vi "环境参数上传.vi"(11 "错误输入（无错误）":errorcluster) -> (15 "error out":errorcluster)   [LabVIEW 2016, in "数据传输系统-04.lvlib"]
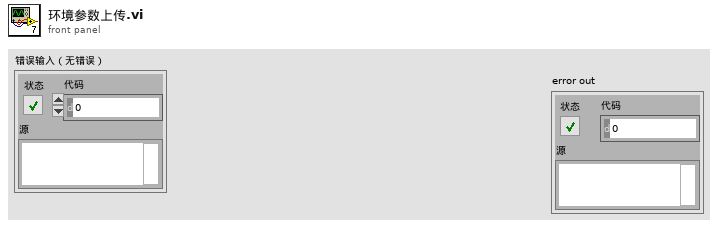
[diagram p1: front panel]
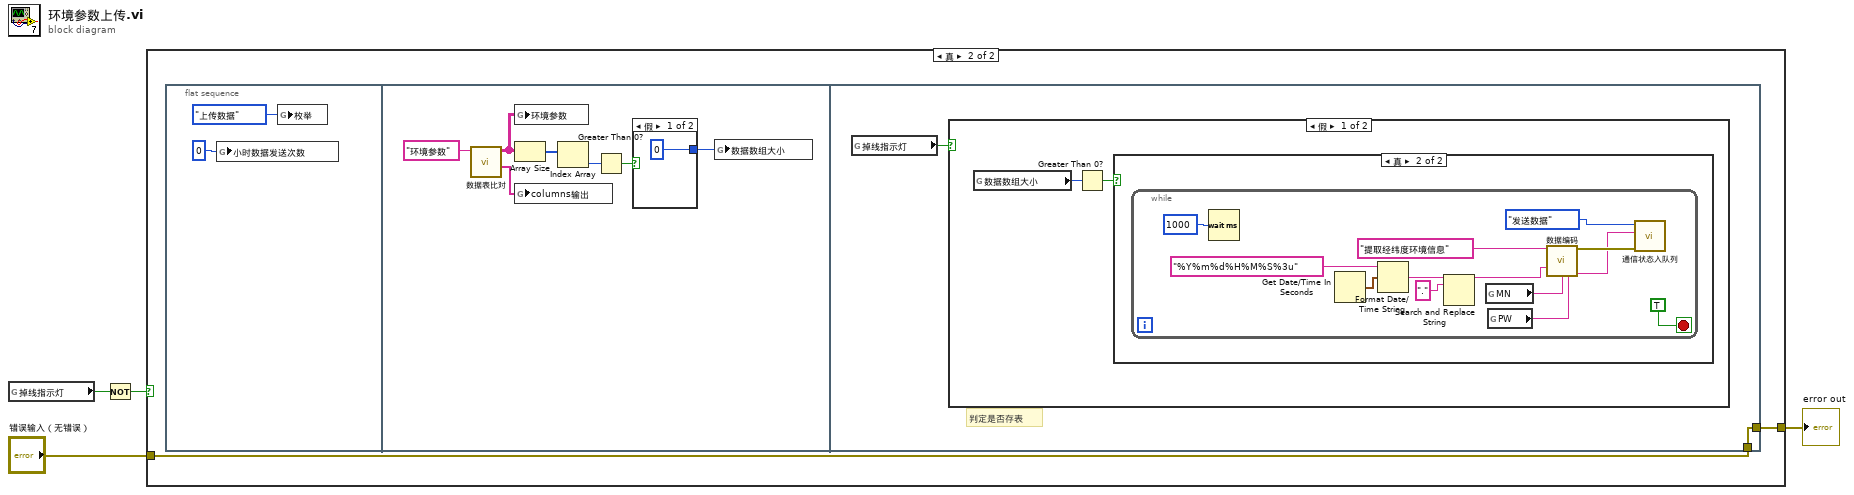
[diagram p0: block diagram]
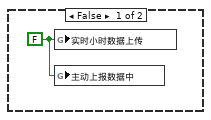
[diagram p2: hidden frame]
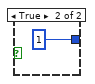
[diagram p3: hidden frame]
diagram:
  n1 = global read "全局 数据发送重叠.vi" "掉线指示灯"() -> (w4:bool)
  n2 = Not(x=w4) -> (.not. x?=w1:bool)
  n3 = case shown="真" w1 {
    tunnel: [_ w6] -> w3
    tunnel: "错误输入（无错误）" -> [_ w7]
    frame False {
      w5 = FALSE ("小时数据上传")
      n4 = global write "全局1.vi" "实时小时数据上传"(w5) -> ()
      n5 = global write "全局 数据发送重叠.vi" "主动上报数据中"(w5) -> ()
    }
    frame True {
      n6 = flat-sequence {
        tunnel: [w19] -> w6
        tunnel: w7 -> [w19]
        frame #0 {
          n7 = global write "全局 小时数据发送次数.vi" "小时数据发送次数"(0 ("小时数据发送次数")) -> ()
          n8 = global write "全局1.vi" "枚举"(enum16{"返回请求应答", "上传数据", "返回执行结果"}."上传数据" ("枚举")) -> ()
        }
        frame #1 {
          n9 = call "数据表比对.vi"("table输入"="环境参数" ("新元素/子数组")) -> ("columns输出"=w16:string[], "待发送数据"=w14:string[][])  [unwired: 7 in, 2 out]
          n10 = global write "全局 环境参数.vi" "环境参数"(w14) -> ()
          n11 = Array Size(array=w14) -> (size(s)=w13:i32[])
          n12 = global write "全局 环境参数.vi" "columns输出"(w16) -> ()
          n13 = Index Array(array=w13) -> (element=w12:i32)  [unwired: 1 in]
          n14 = Greater Than 0?(x=w12) -> (x > 0?=w11:bool)
          n15 = case shown="假" w11 {
            tunnel: [0 ("数据数组大小") 1 ("数据数组大小")] -> w10
            frame False {
            }
            frame True {
            }
          }
          n16 = global write "全局 数据数组大小.vi" "数据数组大小"(w10) -> ()
        }
        frame #2 {
          # "判定是否存表"
          n17 = global read "全局 数据发送重叠.vi" "掉线指示灯"() -> (w20:bool)
          n18 = case shown="假" w20 {
            frame False {
              n19 = global read "全局 数据数组大小.vi" "数据数组大小"() -> (w21:i32)
              n20 = Greater Than 0?(x=w21) -> (x > 0?=w22:bool)
              n21 = case shown="真" w22 {
                frame False {
                }
                frame True {
                  n22 = while {
                    stop <- TRUE stop-if-true
                    n23 = Wait (ms)(milliseconds to wait=u32 1000 ("等待时间（毫秒）")) -> ()  [unwired: 1 out]
                    n24 = Get Date/Time In Seconds() -> (seconds since 1Jan1904=w28:timestamp)
                    n25 = Format Date/Time String(time format string (%c)="%Y%m%d%H%M%S%3u" ("时间格式字符串(%c)"), seconds (now)=w28) -> (date/time string=w27:string)  [unwired: 1 in]
                    n26 = Search and Replace String(input string=w27, search string="." ("搜索字符串")) -> (result string=w25:string)  [unwired: 6 in, 3 out]
                    n27 = global read "断电保存全局.vi" "MN"() -> (w35:string)
                    n28 = global read "断电保存全局.vi" "PW"() -> (w34:string)
                    n29 = call "数据编码.vi"("table输入"="提取经纬度环境信息" ("新元素/子数组"), "QN"=w25, "MN"=w35, "PW"=w34) -> ("错误常量"=w33:errorcluster, "通讯包字符串"=w23:string)  [unwired: 10 in]
                    n30 = call "通信状态入队列.vi"("错误输入（无错误）"=w33, "发送报文"=w23, "枚举"=enum16{"打开连接", "发送数据", "读取数据", "数据处理", "关闭连接"}."发送数据") -> ()  [unwired: 8 in, 1 out]
                  }
                }
              }
            }
            frame True {
            }
          }
        }
      }
    }
  }
  "error out" <- w3
